vi "StartSequenceAcquisition.vi"(8 "error in (no error)":errorcluster, 10 "DataExchange":T1, 11 "Stage in":refnum<class "Stage.lvclass">) -> (0 "error out":errorcluster, 3 "Stage out":refnum<class "Stage.lvclass">)   [LabVIEW 2020]
uses:
  Device/Device/DataExchange.ctl
  Interface/DataListener/DataListener.lvclass
  Stage.lvclass
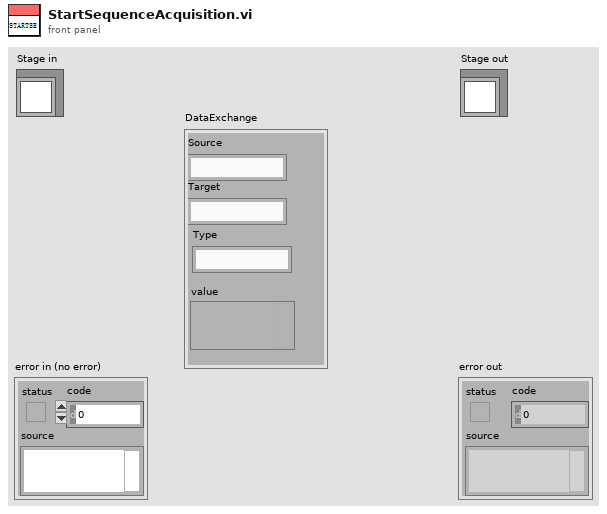
[diagram p1: front panel]
types:
  T1 = typedef "DataListener.lvclass/DataExchange.ctl" = cluster{"Source":string, "Target":string, "Type":string, "value":variant}
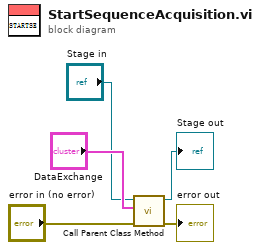
[diagram p0: block diagram]
diagram:
  n1 = call-parent "Call Parent Class Method"("error in (no error)"="error in (no error)", "DataExchange"="DataExchange", "Device in"="Stage in") -> ("error out"=→"error out":errorcluster, "Device out"=→"Stage out":refnum<class "Stage.lvclass">)  [unwired: 7 in]
